vi "getDLLpath.vi"() -> (0 "DLL_Path":path)   [LabVIEW 2018]
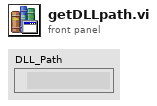
[diagram p1: front panel]
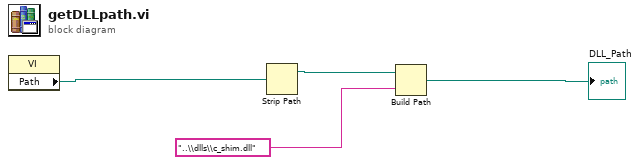
[diagram p0: block diagram]
diagram:
  n1 = property class="VI"() -> ("Path"=w2:path)  [unwired: 2 in, 2 out]
  n2 = Strip Path(path=w2) -> (stripped path=w4:path)  [unwired: 1 out]
  n3 = Build Path(base path=w4, name or relative path="..\\dlls\\c_shim.dll") -> (appended path=→"DLL_Path":path)
